vi "F Dwf Digital Out Counter Set.vi"(7 "vHigh":u32, 8 "error in (no error)":errorcluster, 9 "vLow":u32, 10 "idxChannel":i32, 11 "hdwf":i32) -> (0 "error out":errorcluster, 3 "function return":i32)   [LabVIEW 2019, in "Olasdwf.lvlib"]
doc: "DWFAPI int FDwfDigitalOutCounterSet(HDWF hdwf, int idxChannel, unsigned int vLow, unsigned int vHigh);"
uses:
  Olasdwf.lvlib
  Windows/System32/dwf.dll
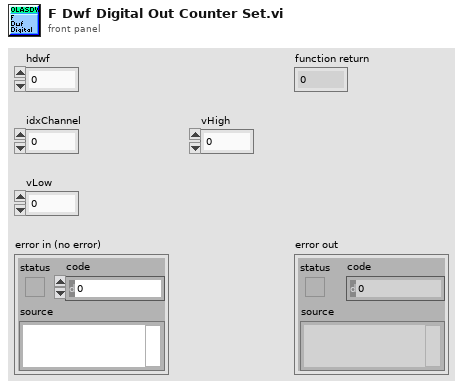
[diagram p1: front panel]
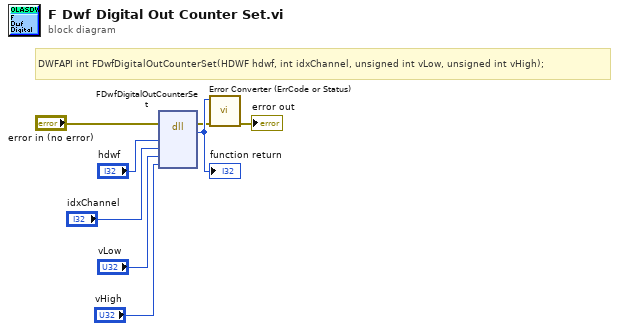
[diagram p0: block diagram]
diagram:
  # "DWFAPI int FDwfDigitalOutCounterSet(HDWF hdwf, int idxChannel, unsigned int vLow, unsigned int vHigh);"
  n1 = dll-call lib="C:/Windows/System32/dwf.*" fn="FDwfDigitalOutCounterSet"(error in="error in (no error)", "hdwf"="hdwf", "idxChannel"="idxChannel", "vLow"="vLow", "vHigh"="vHigh") -> (error out=w2:errorcluster, w8:i32)  [unwired: 6 in, 1 out]
  "function return" <- w8
  n2 = call "Error Converter (ErrCode or Status).vi"("error in (no error)"=w2, "error code"=w8) -> ("error out"=→"error out":errorcluster)  [unwired: 9 in]
